vi "CliGetPGBlockInfo.vi"(0 "ref in":u64, 7 "BlockSize":i32, 9 "var_Block":string, 11 "error in (no error)":errorcluster) -> (1 "Code Date":string, 2 "Interface Date":string, 3 "Author":string, 4 "ref out":u64, 6 "Result":i32, 12 "IntInfo":T1, 13 "Header":string, 14 "Family":string, 15 "error out":errorcluster)   [LabVIEW 2010, in "Snap7.lvlib"]
uses:
  Snap7.lvlib
  windows/lv_snap7.dll
panel:
  in  "var_IntInfo":T1
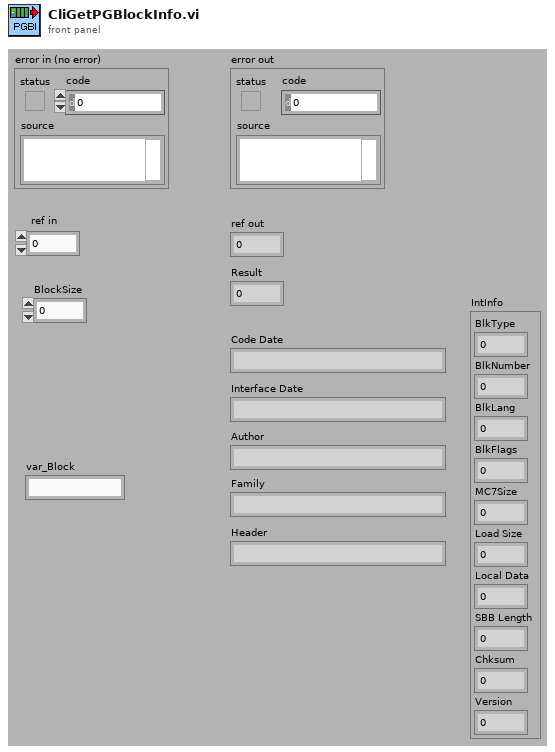
[diagram p1: front panel]
types:
  T1 = cluster{"BlkType":i32, "BlkNumber":i32, "BlkLang":i32, "BlkFlags":i32, "MC7Size":i32, "Load Size":i32, "Local Data":i32, "SBB Length":i32, "Chksum":i32, "Version":i32}
  T2 = enum16{"big-endian, network order", "native, host order", "little-endian"}
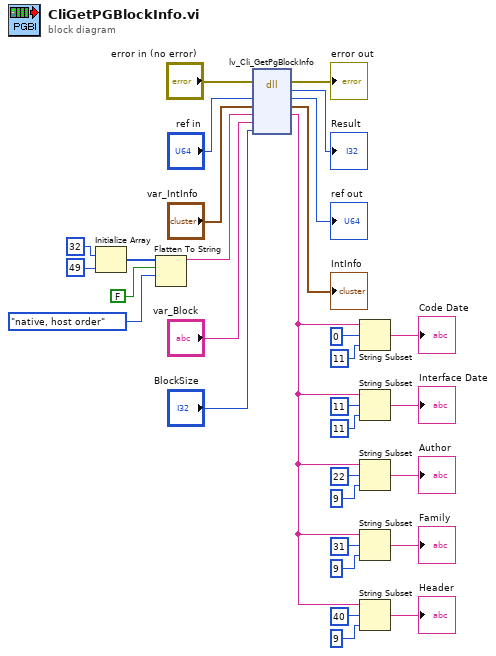
[diagram p0: block diagram]
diagram:
  n1 = Initialize Array(u8 32, 49) -> (w5:u8[])
  n2 = Flatten To String(anything=w5, prepend array or string size? (T)=FALSE, byte order (0:big-endian, network order)=T2."native, host order") -> (data string=w22:string)  [unwired: 1 in, 2 out]
  n3 = dll-call lib="C:/snap7-src-1.0.0/LabVIEW/lib/windows/lv_snap7.dll" fn="lv_Cli_GetPgBlockInfo"(error in="error in (no error)", "Client"="ref in", "var_IntInfo"="var_IntInfo", "var_ChrInfo"=w22, "var_Block"="var_Block", "BlockSize"="BlockSize") -> (error out=→"error out":errorcluster, "return type"=→"Result":i32, "Client"=→"ref out":u64, "var_IntInfo"=→"IntInfo":T1, "var_ChrInfo"=w6:string)  [unwired: 4 in, 1 out]
  n4 = String Subset(string=w6, offset (0)=0, length (rest)=11 ("length (rest)")) -> (substring=→"Code Date":string)
  n5 = String Subset(string=w6, offset (0)=11, length (rest)=11 ("length (rest)")) -> (substring=→"Interface Date":string)
  n6 = String Subset(string=w6, offset (0)=22, length (rest)=9 ("length (rest)")) -> (substring=→"Author":string)
  n7 = String Subset(string=w6, offset (0)=31, length (rest)=9 ("length (rest)")) -> (substring=→"Family":string)
  n8 = String Subset(string=w6, offset (0)=40, length (rest)=9 ("length (rest)")) -> (substring=→"Header":string)
